vi "Teleop Call.vi"(9 "Axes":dbl[](array[numeric]), 10 "Button Values":bool[](array[boolean])) -> ()   [LabVIEW 2017]
uses:
  Implementation/Elevator Operations.ctl
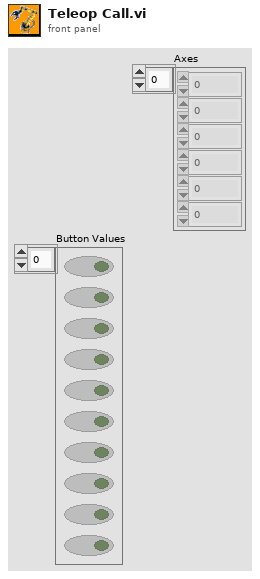
[diagram p1: front panel]
types:
  T1 = enum16{"Hold Position", "Bottom Position", "Top Position"}
  T2 = typedef "Elevator Operations.ctl" = enum16{"Reserve", "Read Current", "Pick Up Cube (Lowest)", "Switch", "Scale", "Immediate"}
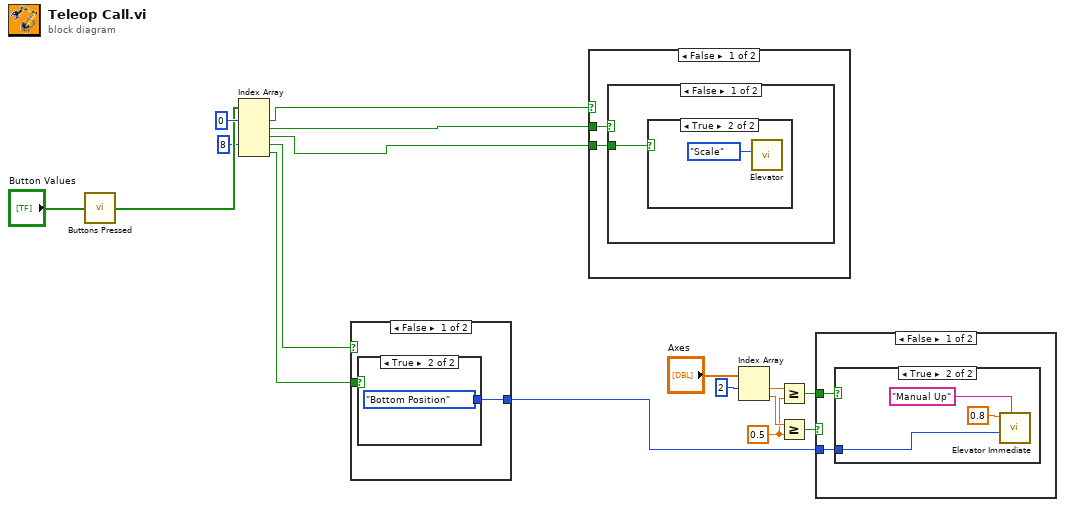
[diagram p0: block diagram]
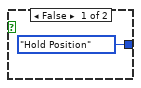
[diagram p2: hidden frame]
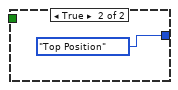
[diagram p3: hidden frame]
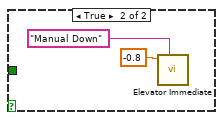
[diagram p5: hidden frame]
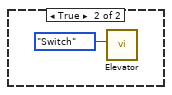
[diagram p7: hidden frame]
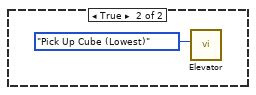
[diagram p8: hidden frame]
diagram:
  w8 = 0.5 ("y")
  n1 = call "Buttons Pressed.vi"("Button Values"="Button Values") -> ("Button Presses"=w16:bool[])
  n2 = Index Array(array=w16, index #1=0 ("index"), index #4=8 ("index")) -> (element #1=w14:bool, element #2=w13:bool, element #3=w5:bool, element #4=w3:bool, element #5=w2:bool)  [unwired: 3 in]
  n3 = case shown="False" w3 {
    tunnel: w2 -> [w19 _]
    tunnel: [w18 T1."Top Position" ("Pneumatic Operation")] -> w1
    frame False {
      n4 = case shown="True" w19 {
        tunnel: [T1."Hold Position" ("Pneumatic Operation") T1."Bottom Position" ("Pneumatic Operation")] -> w18
        frame False {
        }
        frame True {
        }
      }
    }
    frame True {
    }
  }
  n5 = case shown="False" w14 {
    tunnel: w13 -> [w24 _]
    tunnel: w5 -> [w23 _]
    frame False {
      n6 = case shown="False" w24 {
        tunnel: w23 -> [w25 _]
        frame False {
          n7 = case shown="True" w25 {
            frame False {
            }
            frame True {
              n8 = call "Elevator.vi"("Operation"=Elevator_Operations."Scale") -> ()  [unwired: 10 in, 1 out]
            }
          }
        }
        frame True {
          n9 = call "Elevator.vi"("Operation"=Elevator_Operations."Switch") -> ()  [unwired: 10 in, 1 out]
        }
      }
    }
    frame True {
      n10 = call "Elevator.vi"("Operation"=Elevator_Operations."Pick Up Cube (Lowest)") -> ()  [unwired: 10 in, 1 out]
    }
  }
  n11 = Index Array(array="Axes", index #1=2 ("index")) -> (element #1=w10:dbl, element #2=w9:dbl)  [unwired: 1 in]
  n12 = Greater Or Equal?(x=w10, y=w8) -> (x >= y?=w6:bool)
  n13 = Greater Or Equal?(x=w9, y=w8) -> (x >= y?=w7:bool)
  n14 = case shown="False" w7 {
    tunnel: w6 -> [w30 _]
    tunnel: w1 -> [w29 _]
    frame False {
      n15 = case shown="True" w30 {
        tunnel: w29 -> [_ w31]
        frame False {
        }
        frame True {
          n16 = call "Elevator Immediate.vi"("Description"="Manual Up", "Pneumatic Operation"=w31, "Setpoint"=0.8) -> ()  [unwired: 8 in, 1 out]
        }
      }
    }
    frame True {
      n17 = call "Elevator Immediate.vi"("Description"="Manual Down", "Setpoint"=-0.8) -> ()  [unwired: 9 in, 1 out]
    }
  }
